vi "Read CloneRegRef.vi"(8 "error in (no error)":errorcluster, 11 "NistModuleAdmin in":refnum<class "ModuleAdmin.lvclass">) -> (0 "error out":errorcluster, 2 "CloneRegRef":refnum<data-value>, 3 "NistModuleAdmin out":refnum<class "ModuleAdmin.lvclass">)   [LabVIEW 2018, in "ModuleAdmin.lvlib" / "ModuleAdmin.lvclass"]
uses:
  ModuleAdmin.lvclass
  CloneRegistration/CloneRegistration.lvclass
  ModuleAdmin.lvclass/ModuleAdmin.ctl
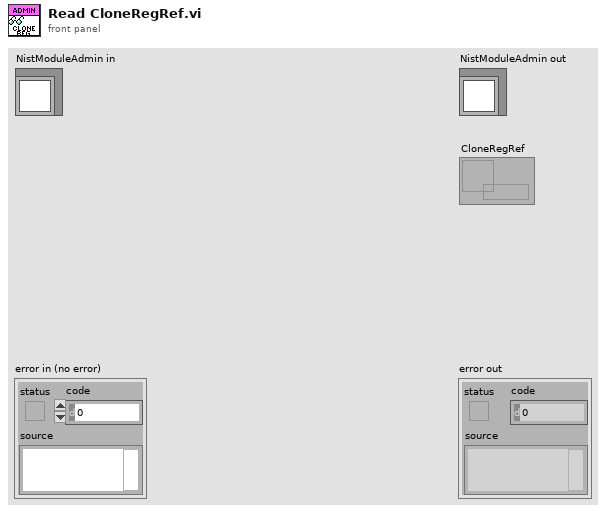
[diagram p1: front panel]
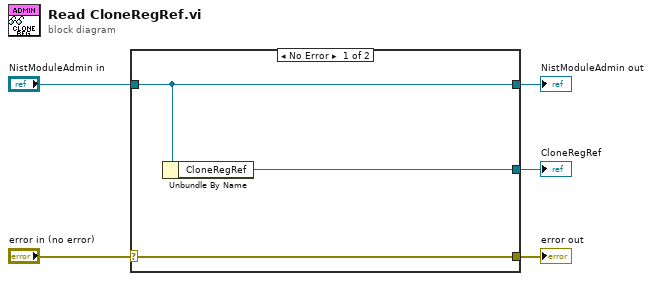
[diagram p0: block diagram]
diagram:
  n1 = case shown="No Error" "error in (no error)" {
    selector: "error in (no error)" -> [w8 w9]
    tunnel: [w8 w9] -> w4
    tunnel: [w7 w10] -> w2
    tunnel: "NistModuleAdmin in" -> [w7 w10]
    tunnel: [w6 _] -> w1
    frame No Error {
      n2 = Unbundle By Name(w7) -> ("CloneRegRef"=w6:refnum<data-value>)
    }
    frame Error {
    }
  }
  "error out" <- w4
  "NistModuleAdmin out" <- w2
  "CloneRegRef" <- w1
